vi "Create Subscription.vi"(7 "Inbound Message":refnum<user-event>, 8 "error in (no error)":errorcluster, 9 "SessionMailbox":refnum<queue>, 10 "QoS":T1, 11 "Topic Filter":string) -> (0 "error out":errorcluster, 3 "Subscription out":refnum<class "Subscription.lvclass">)   [LabVIEW 2013, in "MQTT Server.lvlib" / "Subscription.lvclass"]
uses:
  Subscription.lvclass
  Control Packets/ControlPacket/QualityOfService -- enum.ctl
  MQTT_Base/Response -- cluster.ctl
  Control Packets/ControlPacket/ControlPacket.lvclass
  Control Packets/PUBLISH/PUBLISH.lvclass
  Subscription/Queued Message -- cluster.ctl
  Subscription.lvclass/Subscription.ctl
  process.vi
  TopicFilter/TopicFilter.lvclass
  MQTT_Base/MQTT_Base.lvclass
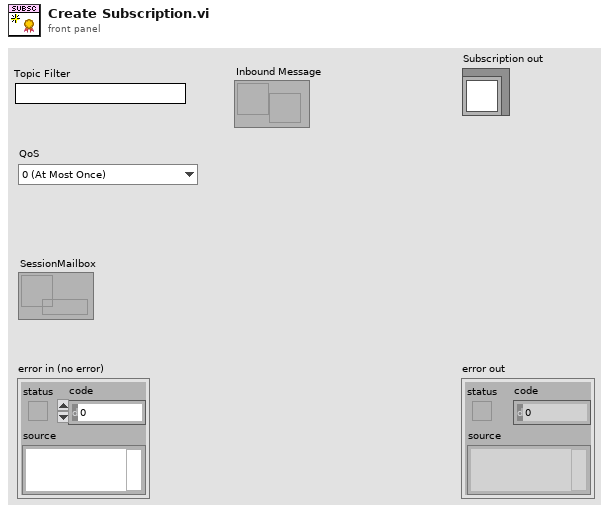
[diagram p1: front panel]
types:
  T1 = typedef "ControlPacket.lvclass/QualityOfService -- enum.ctl" = enum16{"0 (At Most Once)", "1 (At Least Once)", "2 (Exactly Once)"}
  T2 = typedef "MQTT Server.lvlib/Subscription.lvclass/Queued Message -- cluster.ctl" = cluster{"Message":refnum<class "PUBLISH.lvclass">, "PUBREC received":bool}
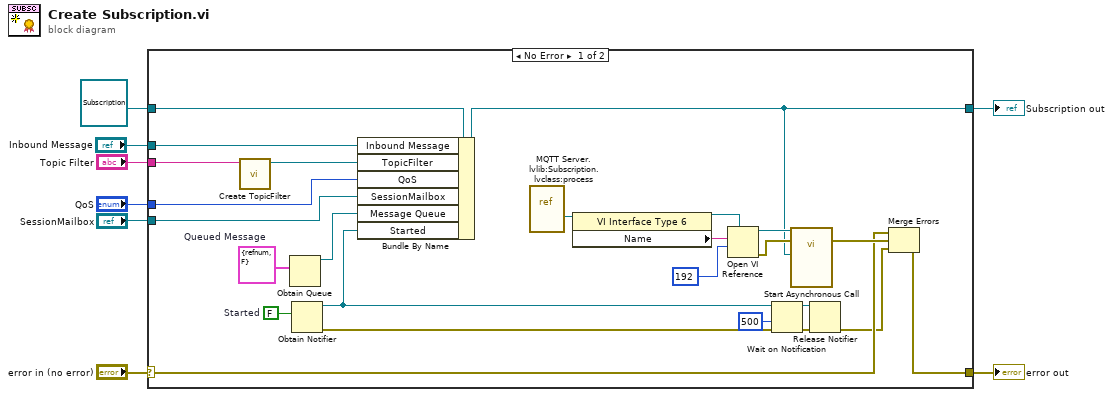
[diagram p0: block diagram]
diagram:
  n1 = case shown="No Error" "error in (no error)" {
    selector: "error in (no error)" -> [w13 w35]
    tunnel: [w11 w35] -> w7
    tunnel: [w14 w34] -> w5
    tunnel: refnum<class "Subscription.lvclass"> refnum ("Subscription in") -> [w31 w34]
    tunnel: "Topic Filter" -> [w10 _]
    tunnel: "QoS" -> [w33 _]
    tunnel: "SessionMailbox" -> [w32 _]
    tunnel: "Inbound Message" -> [w29 _]
    frame No Error {
      w28 = FALSE  # Started
      w30 = T2 {"Message"=refnum, "PUBREC received"=FALSE}  # Queued Message
      n2 = call "Create TopicFilter.vi"("Topic Filter"=w10) -> ("TopicFilter out"=w9:refnum<class "TopicFilter.lvclass">)  [unwired: 9 in, 1 out]
      n3 = Obtain Queue(element data type=w30) -> (queue out=w27:refnum<queue>)  [unwired: 4 in, 2 out]
      n4 = Obtain Notifier(notification data type=w28) -> (notifier out=w26:refnum<notifier>, error out=w23:errorcluster)  [unwired: 3 in, 1 out]
      n5 = Bundle By Name(cluster=w31, "Inbound Message"=w29, "TopicFilter"=w9, "QoS"=w33, "SessionMailbox"=w32, "Message Queue"=w27, "Started"=w26) -> (w14:refnum<class "Subscription.lvclass">)
      n6 = vi-ref "MQTT Server.lvlib:Subscription.lvclass:process.vi"() -> (w21:refnum<vi>)
      n7 = property class="VI Interface Type 6"(reference=w21) -> (reference out=w19:refnum<vi>, "Name"=w20:string)  [unwired: 1 in, 1 out]
      n8 = Open VI Reference(type specifier VI Refnum (for type only)=w19, vi path=w20, options=192) -> (vi reference=w18:refnum<vi>, error out=w17:errorcluster)  [unwired: 3 in]
      n9 = Wait on Notification(notifier=w26, timeout in ms (-1)=500, error in (no error)=w23) -> (notifier out=w24:refnum<notifier>, error out=w22:errorcluster)  [unwired: 1 in, 2 out]
      n10 = call-by-ref "Start Asynchronous Call"(reference=w18, error in=w17, "Subscription in"=w14) -> (error out=w15:errorcluster)  [unwired: 11 in, 1 out]
      n11 = Release Notifier(notifier=w24, error in (no error)=w22) -> (error out=w12:errorcluster)  [unwired: 1 in, 2 out]
      n12 = Merge Errors(w13, w15, w12) -> (w11:errorcluster)
    }
    frame Error {
    }
  }
  "error out" <- w7
  "Subscription out" <- w5
